vi "sweep_type.vi"(8 "error in (no error)":errorcluster, 10 "Sweep Type":string(combo)="Normal", 11 "VISA In":refnum<visa-resource-name>) -> (0 "error out":errorcluster, 3 "VISA Out":refnum<visa-resource-name>)   [LabVIEW 2011]
panel:
  out "String Sent":string
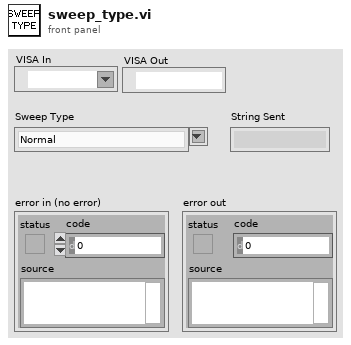
[diagram p1: front panel]
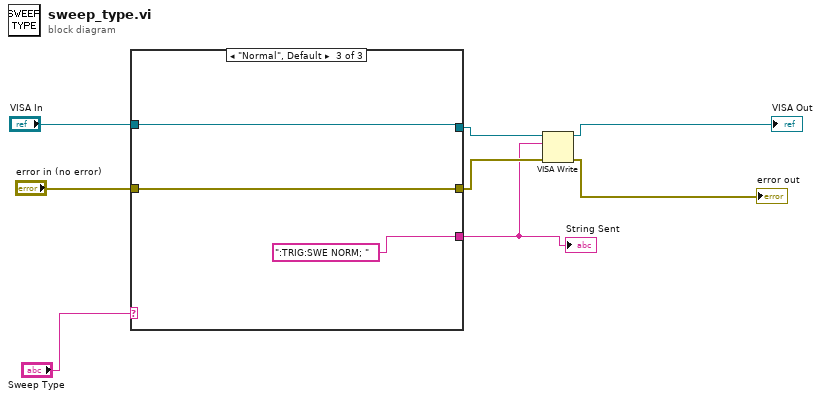
[diagram p0: block diagram]
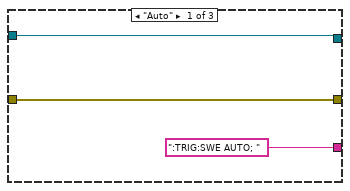
[diagram p2: hidden frame]
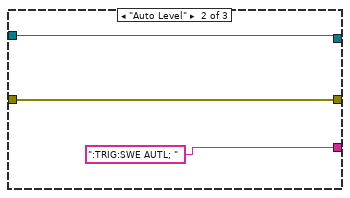
[diagram p3: hidden frame]
diagram:
  n1 = case shown="\"Normal\", Default" "Sweep Type" {
    tunnel: [w11 w14 w17] -> w5
    tunnel: "VISA In" -> [w11 w14 w17]
    tunnel: [w10 w13 w16] -> w4
    tunnel: "error in (no error)" -> [w10 w13 w16]
    tunnel: [":TRIG:SWE AUTO; " ":TRIG:SWE AUTL; " ":TRIG:SWE NORM; "] -> w1
    frame "Auto" {
    }
    frame "Auto Level" {
    }
    frame "Normal", Default {
    }
  }
  "String Sent" <- w1
  n2 = VISA Write(VISA resource name=w5, write buffer=w1, error in (no error)=w4) -> (VISA resource name out=→"VISA Out":refnum<visa-resource-name>, error out=→"error out":errorcluster)  [unwired: 1 out]
